vi "Notifiers Labels.vi"(5 "Instrument":string) -> (0 "Exit String":string, 1 "Ready String":string, 2 "Data String":string, 3 "Status String":string, 4 "Measurement String":string)   [LabVIEW 2014]
panel:
  # "LICENSED MATERIALS – PROPERTY OF IBM\nCopyright IBM Corp. 2016,\nALL RIGHTS RESERVED"
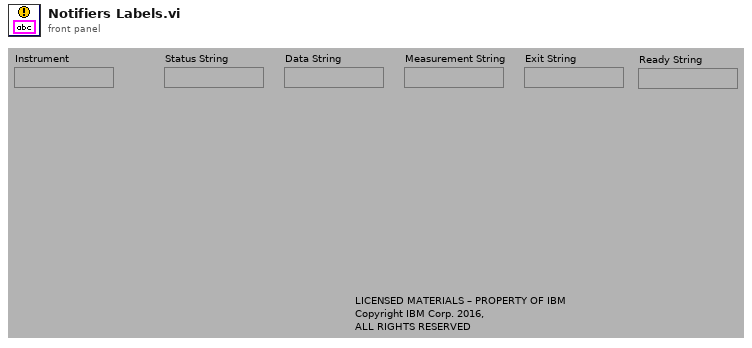
[diagram p1: front panel]
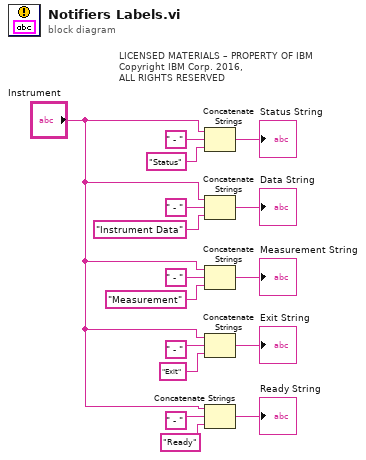
[diagram p0: block diagram]
diagram:
  # "LICENSED MATERIALS – PROPERTY OF IBM\nCopyright IBM Corp. 2016,\nALL RIGHTS RESERVED"
  n1 = Concatenate Strings("Instrument", " - ", "Status") -> (→"Status String":string)
  n2 = Concatenate Strings("Instrument", " - ", "Instrument Data") -> (→"Data String":string)
  n3 = Concatenate Strings("Instrument", " - ", "Measurement") -> (→"Measurement String":string)
  n4 = Concatenate Strings("Instrument", " - ", "Exit") -> (→"Exit String":string)
  n5 = Concatenate Strings("Instrument", " - ", "Ready") -> (→"Ready String":string)
